vi "DriveBaseOpen.vi"(0 "RobotDriveRefnum":string, 1 "DriveBase.lvclass":refnum<class "DriveBase.lvclass">, 5 "Angle Sepoint":dbl, 7 "Angle PID gains":T1, 9 "Velocity PID gains":T1, 11 "Dimensions":cluster{"Wheel Diameter":dbl, "Track Width":dbl}) -> (4 "DriveBase.lvclass 2":refnum<class "DriveBase.lvclass">)   [LabVIEW 2016, in "DriveBase.lvclass"]
uses:
  DriveBase.lvclass
  DriveStates.ctl
  DriveBase.lvclass/DriveBase.ctl
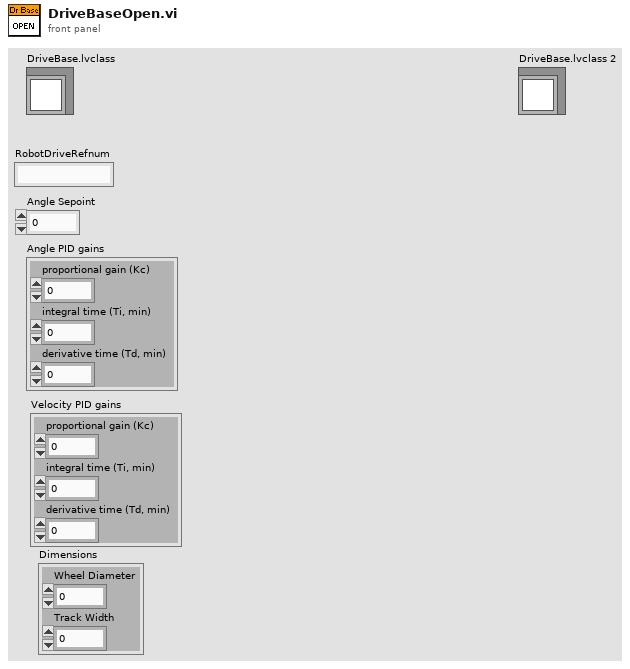
[diagram p1: front panel]
types:
  T1 = cluster{"proportional gain (Kc)":dbl, "integral time (Ti, min)":dbl, "derivative time (Td, min)":dbl}
  T2 = typedef "DriveBase.lvclass/DriveStates.ctl" = enum16{"Tank", "Arcade", "DriveStraight"}
  T3 = cluster{"Right Velocity":dbl, "Left Velocity":dbl, "X Axis Velocity":dbl, "Forward Velocity":dbl}
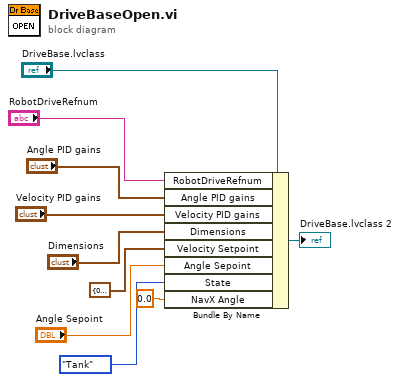
[diagram p0: block diagram]
diagram:
  n1 = Bundle By Name(cluster="DriveBase.lvclass", "RobotDriveRefnum"="RobotDriveRefnum", "Angle PID gains"="Angle PID gains", "Velocity PID gains"="Velocity PID gains", "Dimensions"="Dimensions", "Velocity Setpoint"=T3 {"Right Velocity"=0.0, "Left Velocity"=0.0, "X Axis Velocity"=0.0, "Forward Velocity"=0.0}, "Angle Sepoint"="Angle Sepoint", "State"=DriveStates."Tank", "NavX Angle"=0.0) -> (→"DriveBase.lvclass 2":refnum<class "DriveBase.lvclass">)
